vi "bapsf_motion.vi"(4 "error in":errorcluster, 6 "Request data":variant, 7 "Request":string) -> (0 "error out":errorcluster, 2 "Response data":variant)   [LabVIEW 2022 SP3]
uses:
  typedefs/Device-specific request defs.ctl
panel:
  in  "py interface file":path
  in  "Python session":refnum<k35>
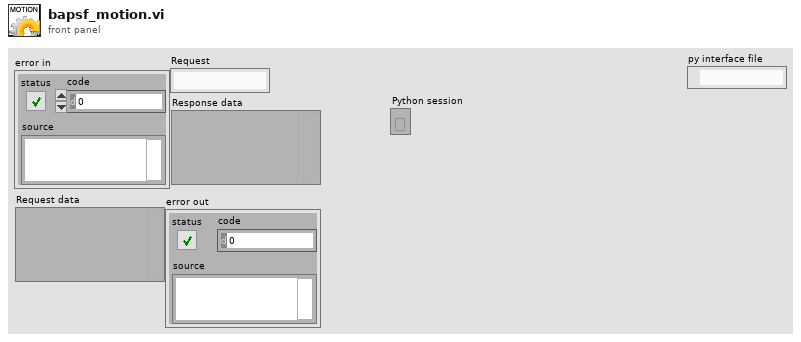
[diagram p1: front panel]
types:
  T1 = typedef "Device-specific request defs.ctl" = cluster{"Request":string, "Key-value types":cluster{"Key":string, "Value type":enum16{"<string>", "<int>"}}[]}[]
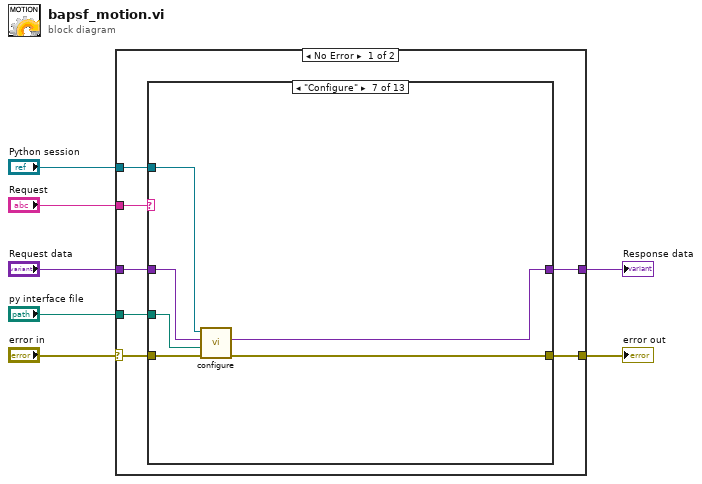
[diagram p0: block diagram]
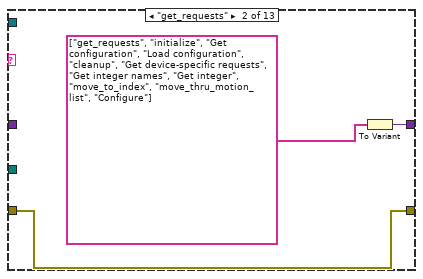
[diagram p3: hidden frame]
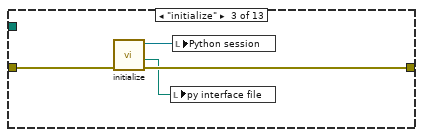
[diagram p4: hidden frame]
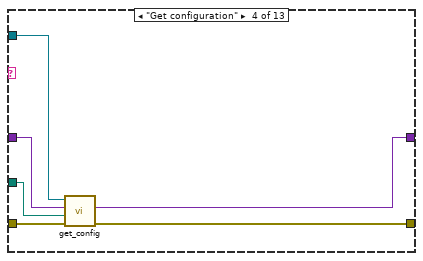
[diagram p5: hidden frame]
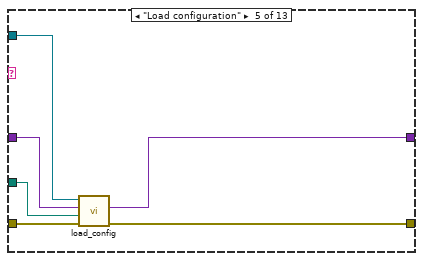
[diagram p6: hidden frame]
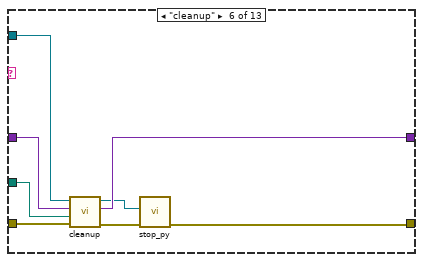
[diagram p7: hidden frame]
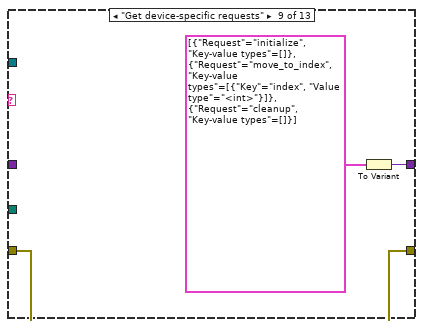
[diagram p9: hidden frame]
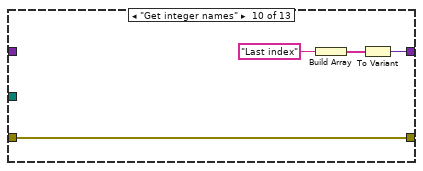
[diagram p10: hidden frame]
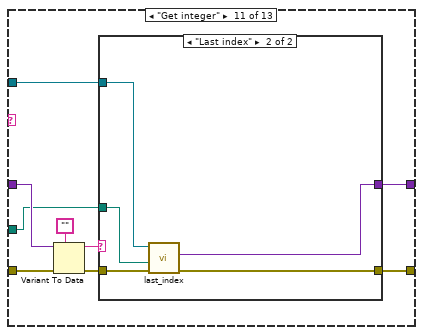
[diagram p11: hidden frame]
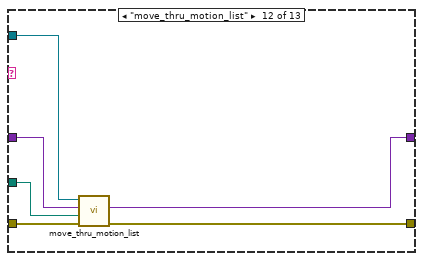
[diagram p13: hidden frame]
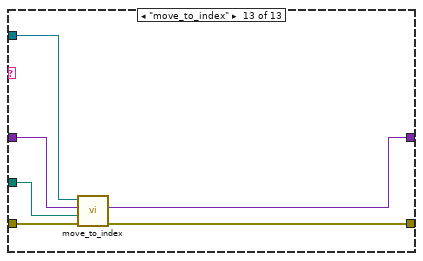
[diagram p14: hidden frame]
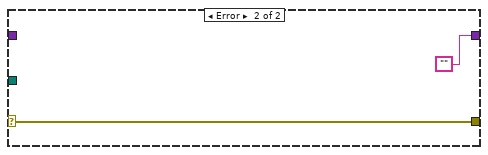
[diagram p15: hidden frame]
diagram:
  n1 = case shown="No Error" "error in" {
    selector: "error in" -> [w13 w87]
    tunnel: [w11 w87] -> w6
    tunnel: "Request" -> [w14 _]
    tunnel: "Request data" -> [w12 _]
    tunnel: [w10 ""] -> w3
    tunnel: "Python session" -> [w9 _]
    tunnel: "py interface file" -> [w8 _]
    frame No Error {
      n2 = case shown="\"Configure\"" w14 {
        tunnel: w13 -> [w16 w19 w22 w29 w35 w43 w49 w51 w52 w58 w67 w79 w85]
        tunnel: w12 -> [w15 _ _ w28 w33 w41 w47 w50 _ _ w66 w77 w83]
        tunnel: [w16 w19 w23 w27 w31 w37 w48 w51 w52 w58 w61 w75 w81] -> w11
        tunnel: [w15 w18 _ w26 w30 w39 w44 w50 w53 w55 w59 w74 w80] -> w10
        tunnel: w9 -> [_ _ _ w25 w32 w40 w45 _ _ _ w62 w76 w82]
        tunnel: w8 -> [_ _ _ w24 w34 w42 w46 _ _ _ w60 w78 w84]
        frame "", Default {
        }
        frame "get_requests" {
          n3 = To Variant(anything=string[] ["get_requests", "initialize", "Get configuration", "Load configuration", "cleanup", "Get device-specific requests", "Get integer names", "Get integer", "move_to_index", "move_thru_motion_list", "Configure"]) -> (Variant=w18:variant)
        }
        frame "initialize" {
          n4 = call "initialize.vi"("error in (no error)"=w22) -> ("error out"=w23:errorcluster, "py interface file"=w21:path, "Python session out"=w20:refnum<k35>)  [unwired: 4 in]
          n5 = local write "py interface file"(w21) -> ()
          n6 = local write "Python session"(w20) -> ()
        }
        frame "Get configuration" {
          n7 = call "get_config.vi"("error in (no error)"=w29, "py interface file"=w24, "Request data"=w28, "Python session in"=w25) -> ("error out"=w27:errorcluster, "Response data"=w26:variant)  [unwired: 1 in, 1 out]
        }
        frame "Load configuration" {
          n8 = call "load_config.vi"("error in (no error)"=w35, "py interface file"=w34, "Request data"=w33, "Python session in"=w32) -> ("error out"=w31:errorcluster, "Response data"=w30:variant)  [unwired: 1 in, 1 out]
        }
        frame "cleanup" {
          n9 = call "cleanup.vi"("error in (no error)"=w43, "py interface file"=w42, "Request data"=w41, "Python session in"=w40) -> ("error out"=w38:errorcluster, "Response data"=w39:variant, "Python session out"=w36:refnum<k35>)  [unwired: 1 in]
          n10 = call "stop_py.vi"("error in"=w38, "Python session"=w36) -> ("error out"=w37:errorcluster)  [unwired: 5 in]
        }
        frame "Configure" {
          n11 = call "configure.vi"("error in (no error)"=w49, "py interface file"=w46, "Request data"=w47, "Python session in"=w45) -> ("error out"=w48:errorcluster, "Response data"=w44:variant)  [unwired: 1 in, 1 out]
        }
        frame "Get run-time state" {
        }
        frame "Get device-specific requests" {
          n12 = To Variant(anything=T1 [{"Request"="initialize", "Key-value types"=[]}, {"Request"="move_to_index", "Key-value types"=[{"Key"="index", "Value type"=enum."<int>"}]}, {"Request"="cleanup", "Key-value types"=[]}] ("Device-specific request defs")) -> (Variant=w53:variant)
        }
        frame "Get integer names" {
          n13 = Build Array("Last index") -> (w57:string[])
          n14 = To Variant(anything=w57) -> (Variant=w55:variant)
        }
        frame "Get integer" {
          n15 = Variant To Data(error in=w67, type="", Variant=w66) -> (data=w64:string, error out=w63:errorcluster)
          n16 = case shown="\"Last index\"" w64 {
            tunnel: w63 -> [w68 w73]
            tunnel: w62 -> [_ w71]
            tunnel: [w68 w70] -> w61
            tunnel: w60 -> [_ w72]
            tunnel: [_ w69] -> w59
            frame "", Default {
            }
            frame "Last index" {
              n17 = call "last_index.vi"("error in (no error)"=w73, "py interface file"=w72, "Python session in"=w71) -> ("error out"=w70:errorcluster, "Response data"=w69:variant)  [unwired: 2 in, 1 out]
            }
          }
        }
        frame "move_thru_motion_list" {
          n18 = call "move_thru_motion_list.vi"("error in (no error)"=w79, "py interface file"=w78, "Request data"=w77, "Python session in"=w76) -> ("error out"=w75:errorcluster, "Response data"=w74:variant)  [unwired: 1 in, 1 out]
        }
        frame "move_to_index" {
          n19 = call "move_to_index.vi"("error in (no error)"=w85, "py interface file"=w84, "Request data"=w83, "Python session in"=w82) -> ("error out"=w81:errorcluster, "Response data"=w80:variant)  [unwired: 1 in, 1 out]
        }
      }
    }
    frame Error {
    }
  }
  "Response data" <- w3
  "error out" <- w6
